vi "communication.vi"(8 "error in (no error)":errorcluster, 11 "VISA resource name":refnum<visa-resource-name>) -> (0 "error out":errorcluster, 3 "VISA resource name out":refnum<visa-resource-name>)   [LabVIEW 2020]
panel:
  in  "Command input":T1={"Start meas"=33, "Command"="Reset carriage", "Length"=1, "Payload"=1} {"Start meas" max=1}
  out "read buffer":string
  out "return count":u32
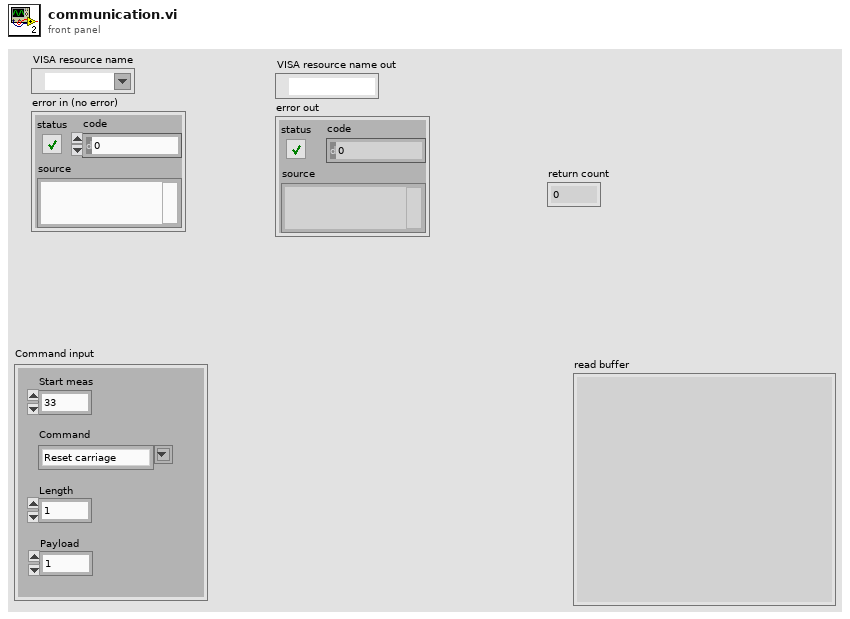
[diagram p1: front panel]
types:
  T1 = cluster{"Start meas":u8, "Command":string, "Length":u8, "Payload":u8}
  T2 = cluster{"VISA resource name out":refnum<visa-resource-name>, "error out":errorcluster}
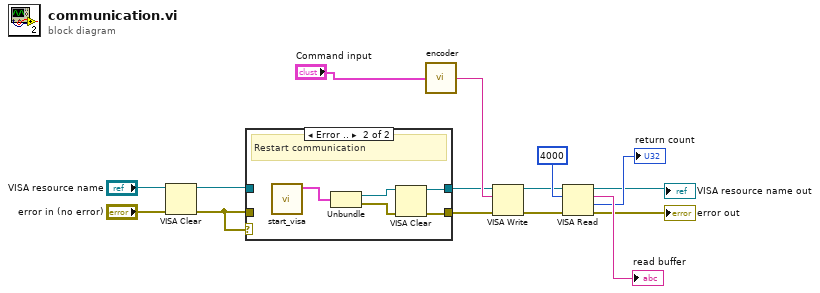
[diagram p0: block diagram]
diagram:
  n1 = VISA Clear(VISA resource name="VISA resource name", error in (no error)="error in (no error)") -> (VISA resource name out=w5:refnum<visa-resource-name>, error out=w4:errorcluster)
  n2 = case shown="Error .." w4 {
    tunnel: w5 -> [w17 _]
    tunnel: w4 -> [w16 _]
    tunnel: [w17 w21] -> w7
    tunnel: [w16 w20] -> w6
    frame No Error {
    }
    frame Error {
      # "Restart communication"
      n3 = call "start_visa.vi"() -> ("output cluster"=w22:T2)  [unwired: 11 in]
      n4 = Unbundle(w22) -> ("VISA resource name out"=w19:refnum<visa-resource-name>, "error out"=w18:errorcluster)
      n5 = VISA Clear(VISA resource name=w19, error in (no error)=w18) -> (VISA resource name out=w21:refnum<visa-resource-name>, error out=w20:errorcluster)
    }
  }
  n6 = call "encoder.vi"("Command input"="Command input") -> ("Command string"=w14:string)
  n7 = VISA Write(VISA resource name=w7, write buffer=w14, error in (no error)=w6) -> (VISA resource name out=w11:refnum<visa-resource-name>, error out=w13:errorcluster)  [unwired: 1 out]
  n8 = VISA Read(VISA resource name=w11, byte count=u32 4000, error in (no error)=w13) -> (VISA resource name out=→"VISA resource name out":refnum<visa-resource-name>, read buffer=→"read buffer":string, return count=→"return count":u32, error out=→"error out":errorcluster)
